vi "Get All Items By Index.vi"(8 "error in (no error)":errorcluster caption="错误输入（无错误）", 11 "ArrayListClass 输入":refnum<class "ArrayListClass.lvclass"> caption="DNL_LabVIEW Object in") -> (0 "error out":errorcluster caption="错误输出", 2 "Items":variant[](array[variant]), 3 "ArrayListClass 输出":refnum<class "ArrayListClass.lvclass"> caption="DNL_LabVIEW Object out")   [LabVIEW 2012, in "ArrayListClass.lvclass"]
uses:
  ArrayListClass.lvclass
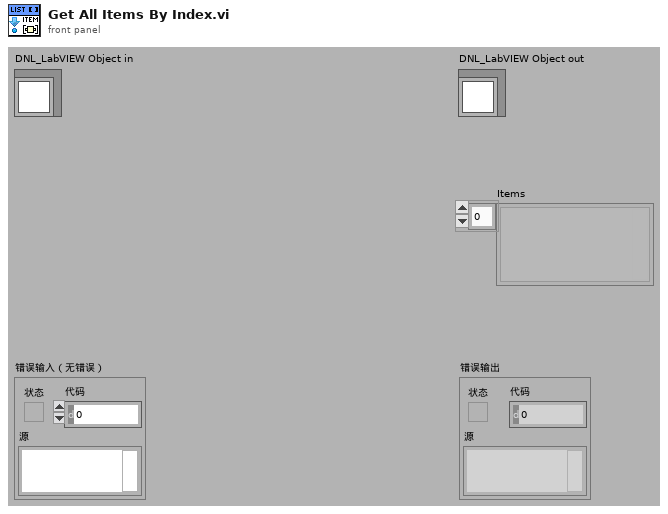
[diagram p1: front panel]
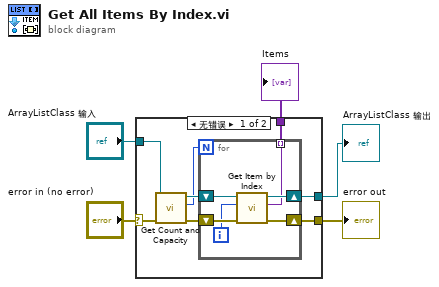
[diagram p0: block diagram]
diagram:
  n1 = case shown="无错误" "error in (no error)" {
    selector: "error in (no error)" -> [w7 w21]
    tunnel: [w8 w21] -> w4
    tunnel: [w11 w20] -> w2
    tunnel: "ArrayListClass 输入" -> [w13 w20]
    tunnel: [w9 _] -> w1
    frame No Error {
      n2 = call "Get Count and Capacity.vi"("error in (no error)"=w7, "ArrayListClass 输入"=w13) -> ("error out"=w10:errorcluster, "Count"=w6:i32, "ArrayListClass 输出"=w12:refnum<class "ArrayListClass.lvclass">)  [unwired: 6 in, 1 out]
      n3 = for {
        N: w6 -> [_]
        shift-right: [w16] -> w11
        shift-left: w12 -> [w17]
        shift-right: [w18] -> w8
        shift-left: w10 -> [w19]
        tunnel: [w15] -> w9 mode=indexing
        i -> [w14]
        n4 = call "Get Item by Index.vi"("error in (no error)"=w19, "index"=w14, "ArrayListClass 输入"=w17) -> ("error out"=w18:errorcluster, "Value"=w15:variant, "ArrayListClass 输出"=w16:refnum<class "ArrayListClass.lvclass">)  [unwired: 6 in]
      }
    }
    frame Error {
    }
  }
  "error out" <- w4
  "ArrayListClass 输出" <- w2
  "Items" <- w1
